vi "Get ATM Message.vi"(8 "error in (no error)":errorcluster, 10 "Tokens":cluster{"Name":string, "Value":string}[](array[cluster]), 11 "Message":string) -> (0 "error out":errorcluster, 3 "String":string)   [LabVIEW 8.6]
doc: "This VI accesses and parses a message string for user display. It provides encapsulation of the core defined messages, so the message set can be updated/modified without having to change this function or any of its callers."
uses:
  Controls/Messages.ctl
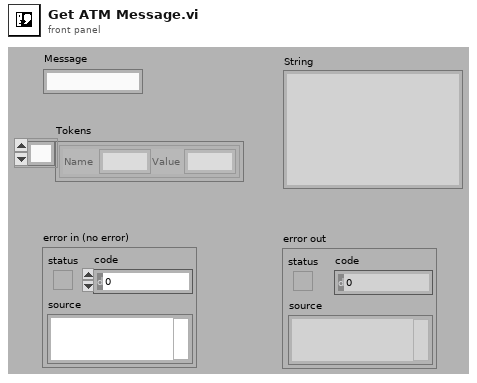
[diagram p1: front panel]
types:
  T1 = typedef "Messages.ctl" = string[][]
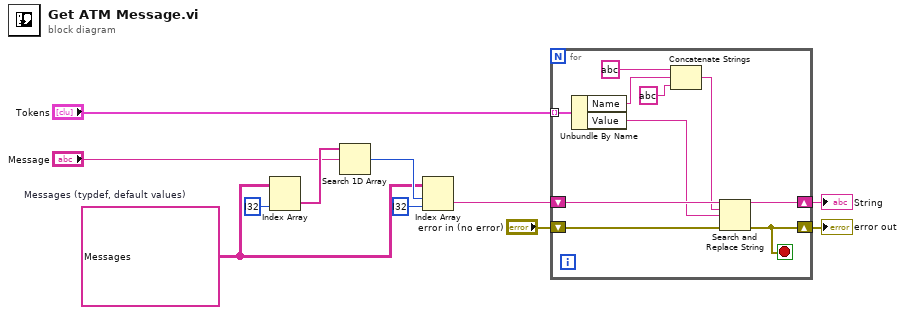
[diagram p0: block diagram]
diagram:
  w1 = T1 ?  # Messages (typdef, default values)
  n1 = Index Array(array=w1, index (col)=i32 ? ("disabled index (col)")) -> (element=w10:string[])  [unwired: 1 in]
  n2 = Search 1D Array(1D array=w10, element="Message") -> (index of element=w7:i32)  [unwired: 1 in]
  n3 = Index Array(array=w1, index (row)=w7, index (col)=i32 ? ("disabled index (col)")) -> (element=w5:string)
  n4 = for {
    tunnel: "Tokens" -> [w21] mode=indexing
    shift-right: [w17] -> w4
    shift-left: "error in (no error)" -> [w18]
    shift-right: [w16] -> w2
    shift-left: w5 -> [w20]
    stop <- w17 stop-if-true
    n5 = Unbundle By Name(w21) -> ("Name"=w15:string, "Value"=w19:string)
    n6 = Concatenate Strings(string ?, w15, string ?) -> (w12:string)
    n7 = Search and Replace String(input string=w20, search string=w12, replace string=w19, error in=w18) -> (result string=w16:string, error out=w17:errorcluster)  [unwired: 4 in, 2 out]
  }
  "error out" <- w4
  "String" <- w2
